vi "1D Array Sum.vi"() -> ()   [LabVIEW 2015]
panel:
  in  "Tab Control":enum32{"Page 1", "Page 2"}(tab)
  out "Array":i32[](array[numeric])
  out "Sum":i32
  # "1D Array Sum"
  # "Pardeep Kumar"
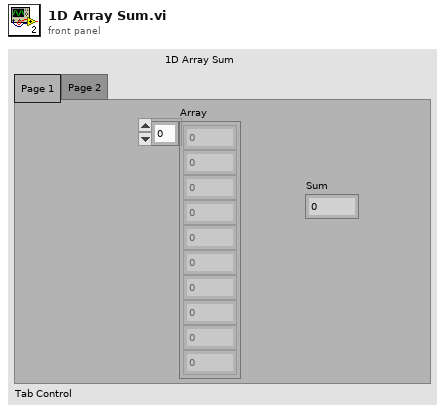
[diagram p1: front panel]
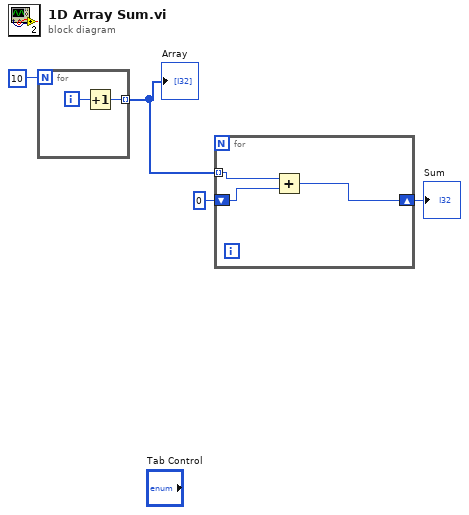
[diagram p0: block diagram]
diagram:
  n1 = for {
    N: 10 -> [_]
    tunnel: [w5] -> w3 mode=indexing
    i -> [w6]
    n2 = Increment(x=w6) -> (x+1=w5:i32)
  }
  "Array" <- w3
  n3 = for {
    tunnel: w3 -> [w9] mode=indexing
    shift-right: [w8] -> w1
    shift-left: 0 -> [w7]
    n4 = Add(x=w9, y=w7) -> (x+y=w8:i32)
  }
  "Sum" <- w1
